vi "Evaluate Wait.vi"(8 "error in (no error)":errorcluster, 11 "Wait in":refnum<class "Wait.lvclass">) -> (0 "error out":errorcluster, 3 "Wait out":refnum<class "Wait.lvclass">)   [LabVIEW 2019, in "Wait.lvclass"]
uses:
  <vilib>/gpm_packages/@cs/Car-wash/Source/Process Steps/Wait/Wait.lvclass
  C:/Program Files/National Instruments/LabVIEW 2019/vi.lib/gpm_packages/@cs/mva-core/Source/IModel/IModel/IModel.lvclass
  C:/Program Files/National Instruments/LabVIEW 2019/vi.lib/ActorFramework/Actor/Actor.lvclass
  <vilib>/gpm_packages/@cs/Car-wash/Source/Process Steps/Wait/Wait.lvclass/Wait.ctl
  <vilib>/gpm_packages/@cs/mva-core/Source/IObserver/IObserver/IObserver.lvclass/IObserver.ctl
  <vilib>/gpm_packages/@cs/mva-core/Source/IModel/IModel/IModel.lvclass/IModel.ctl
  <vilib>/gpm_packages/@cs/mva-core/Source/IMediator/PublishRequest/PublishRequest.lvclass/PublishRequest.ctl
  <vilib>/gpm_packages/@cs/mva-core/Source/IMediator/IMediator Messages/Publish Msg/Publish Msg.lvclass/Publish Msg.ctl
  <vilib>/gpm_packages/@cs/actor-framework-messages/Source/RoundTripMessage/RoundTripMessage.lvclass/RoundTripMessage.ctl
  <vilib>/ActorFramework/Message Enqueuer/Message Enqueuer.lvclass/Message Enqueuer.ctl
  <vilib>/ActorFramework/Time-Delayed Send Message/Time-Delay Override Options.ctl
  <vilib>/ActorFramework/Actor/Actor.lvclass/Actor.ctl
  <vilib>/gpm_packages/@cs/mva-core/Source/IMediator/IMediator Messages/Publish Msg/Send Pre-Addressed Publish.vi
  <vilib>/gpm_packages/@cs/mva-core/Source/IObserver/IObserver/Read Unique ID.vi
  <vilib>/gpm_packages/@cs/mva-core/Source/IMediator/PublishRequest/Pack Publish Request.vi
  <vilib>/ActorFramework/Message Enqueuer/Init from Existing Queue.vi
  <vilib>/ActorFramework/Message Enqueuer/Enqueue.vi
  <vilib>/gpm_packages/@cs/actor-framework-messages/Source/RoundTripMessage/Return Round-Trip Message.vi
  <vilib>/gpm_packages/@cs/mva-core/Source/IModel/IModel/IModel.lvclass
  C:/Program Files/National Instruments/LabVIEW 2019/vi.lib/gpm_packages/@cs/mva-core/Source/IObserver/IObserver/IObserver.lvclass
  <vilib>/gpm_packages/@cs/mva-core/Source/IMediator/IMediator Messages/Publish Msg/Publish Msg.lvclass
  C:/Program Files/National Instruments/LabVIEW 2019/vi.lib/gpm_packages/@cs/actor-framework-messages/Source/RoundTripMessage/RoundTripMessage.lvclass
  <vilib>/gpm_packages/@cs/actor-framework-messages/Source/RoundTripMessage/RoundTripMessage.lvclass
  C:/Program Files/National Instruments/LabVIEW 2019/vi.lib/ActorFramework/Message/Message.lvclass
  <vilib>/ActorFramework/Stop Msg/Stop Msg.lvclass
  <vilib>/Utility/error.llb/Error Cluster From Error Code.vi
  <vilib>/ActorFramework/Message Priority Queue/Priority Enqueue.vi
  <vilib>/gpm_packages/@cs/mva-core/Source/IMediator/PublishRequest/PublishRequest.lvclass
  <vilib>/ActorFramework/Message Enqueuer/Message Enqueuer.lvclass
  <vilib>/ActorFramework/Actor/Actor.lvclass
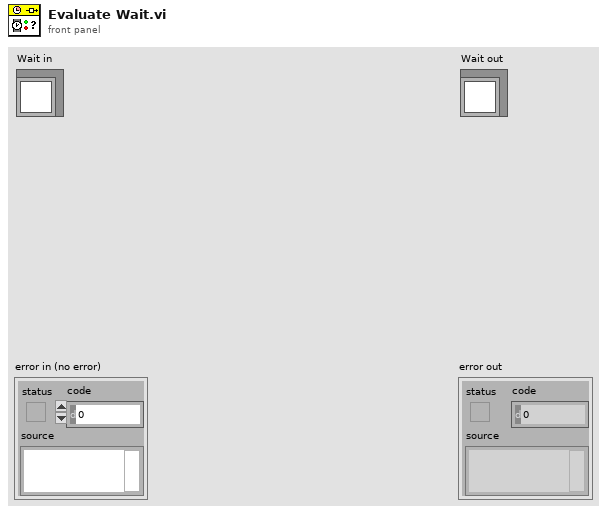
[diagram p1: front panel]
types:
  T1 = typedef "Time-Delay Override Options.ctl" = enum16{"Send next copy now", "Skip next scheduled copy", "Send next copy now and stop all further copies", "Stop all further copies"}
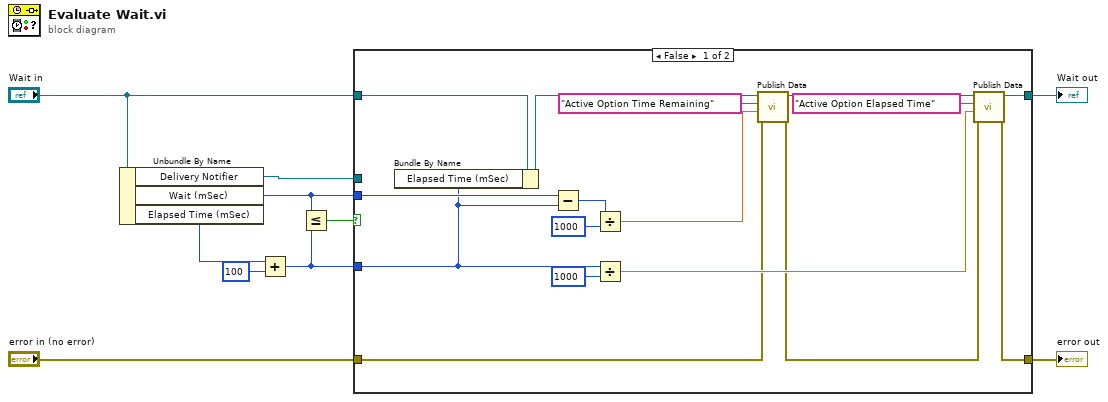
[diagram p0: block diagram]
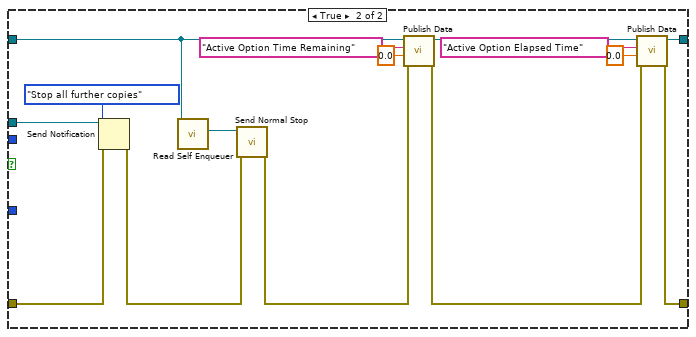
[diagram p2: hidden frame]
diagram:
  n1 = Unbundle By Name("Wait in") -> ("Delivery Notifier"=w3:refnum<notifier>, "Wait (mSec)"=w1:i32, "Elapsed Time (mSec)"=w10:i32)
  n2 = Add(x=w10, y=100) -> (x+y=w2:i32)
  n3 = Less Or Equal?(x=w1, y=w2) -> (x <= y?=w8:bool)
  n4 = case shown="False" w8 {
    tunnel: [w25 w35] -> w6
    tunnel: "Wait in" -> [w26 w31]
    tunnel: [w23 w34] -> w4
    tunnel: "error in (no error)" -> [w14 w38]
    tunnel: w3 -> [_ w40]
    tunnel: w2 -> [w21 _]
    tunnel: w1 -> [w22 _]
    frame False {
      n5 = Bundle By Name(cluster=w26, "Elapsed Time (mSec)"=w21) -> (w12:refnum<class "Wait.lvclass">)
      n6 = Subtract(x=w22, y=w21) -> (x-y=w16:i32)
      n7 = Divide(x=w16, y=1000) -> (x/y=w15:dbl)
      n8 = Divide(x=w21, y=1000) -> (x/y=w19:dbl)
      n9 = call <vilib>:"Publish Data.vi"("error in (no error)"=w14, "Data to Publish"=w15, "Datum Name"="Active Option Time Remaining", "IModel in"=w12) -> ("error out"=w13:errorcluster, "IModel out"=w11:refnum<class "Wait.lvclass">)  [unwired: 6 in]
      n10 = call <vilib>:"Publish Data.vi"("error in (no error)"=w13, "Data to Publish"=w19, "Datum Name"="Active Option Elapsed Time", "IModel in"=w11) -> ("error out"=w23:errorcluster, "IModel out"=w25:refnum<class "Wait.lvclass">)  [unwired: 6 in]
    }
    frame True {
      n11 = Send Notification(notification=Time-Delay_Override_Options."Stop all further copies", notifier=w40, error in (no error)=w38) -> (error out=w37:errorcluster)  [unwired: 1 out]
      n12 = call <vilib>:"Read Self Enqueuer.vi"("Actor"=w31) -> ("Self Enqueuer"=w41:refnum<class "Message Enqueuer.lvclass">)  [unwired: 10 in]
      n13 = call <vilib>:"Send Normal Stop.vi"("error in (no error)"=w37, "Message Enqueuer"=w41) -> ("error out"=w29:errorcluster)  [unwired: 9 in]
      n14 = call <vilib>:"Publish Data.vi"("error in (no error)"=w29, "Data to Publish"=0.0, "Datum Name"="Active Option Time Remaining", "IModel in"=w31) -> ("error out"=w28:errorcluster, "IModel out"=w30:refnum<class "Wait.lvclass">)  [unwired: 6 in]
      n15 = call <vilib>:"Publish Data.vi"("error in (no error)"=w28, "Data to Publish"=0.0, "Datum Name"="Active Option Elapsed Time", "IModel in"=w30) -> ("error out"=w34:errorcluster, "IModel out"=w35:refnum<class "Wait.lvclass">)  [unwired: 6 in]
    }
  }
  "error out" <- w4
  "Wait out" <- w6
